vi "LINX - Photocell_to water level.vi"(8 "AI Channel":u8, 11 "Serial Port":refnum<visa-resource-name>) -> (0 "Photocell Value":u8(slide) scale=0.0..15.0)   [LabVIEW 2020]
doc: "Measure light intensity using a photocell."
uses:
  <vilib>/MakerHub/LINX/Public/Utilities/Open Serial.vi
  <vilib>/MakerHub/LINX/LMH-LINX.lvlib
panel:
  out "Loop Rate (Hz)":u32
  in  "Stop Button":bool
  # "Circuit Schematic"
  # "LINX Device Settings"
  # "Photocell Value"
  # "Photocell Example (Serial Interface)\n\nThis example demonstrates how to measure light intensity using a photocell.\n\nInstructions\n1. Select the COM Port associated with the LINX Device.\n2. Select the Analog Channel connected to the photocell.\n3. Click the Run Arrow."
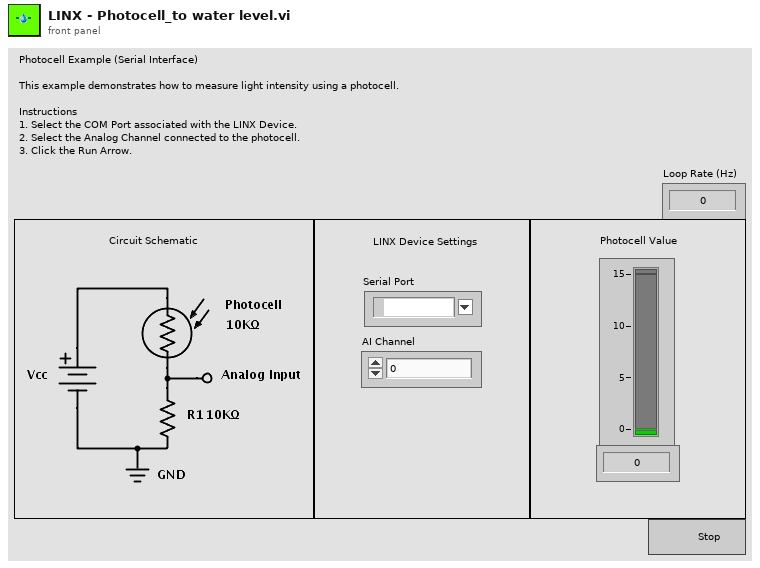
[diagram p1: front panel]
types:
  T1 = typedef "LMH-LINX.lvlib/LINX Ref.ctl" = cluster{"IO":T2, "Interface":T3, "LINX Device Config":T4}
  T2 = typedef "LMH-LINX.lvlib/Platform.ctl" = enum16{"Remote", "Local"}
  T3 = typedef "LMH-LINX.lvlib/Interface.ctl" = enum16{"Serial", "TCP"}
  T4 = typedef "LMH-LINX.lvlib/Device.lvlib/LINX Device Config.ctl" = cluster{"Interface":T3, "COM Port":refnum<visa-resource-name>, "TCP Configuration":T5, "Device Family":u8, "Device ID":u8, "Device Name":string, "TCP Ref":refnum<k5>, "Channels":T6}
  T5 = typedef "LMH-LINX.lvlib/Device.lvlib/TCP Config.ctl" = cluster{"IP Address":string, "Port":u16}
  T6 = typedef "LMH-LINX.lvlib/Channels.ctl" = cluster{"DI":u8[], "DO":u8[], "AI":u8[], "AO":u8[], "PWM":u8[], "QE":u8[], "UART":u8[], "I2C 2":u8[], "SPI":u8[], "CAN":u8[], "Servo":u8[], "AI Ref (V)":dbl, "AI Resolution (Bits)":u8, "AO Ref (V)":dbl, "AO Resolution (Bits)":u8}
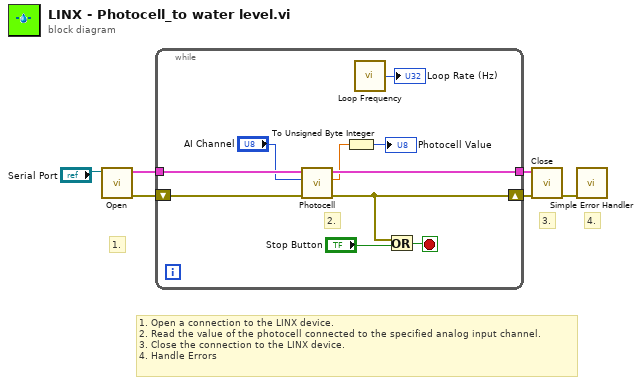
[diagram p0: block diagram]
diagram:
  # "1. Open a connection to the LINX device.\n2. Read the value of the photocell connected to the specified analog input channel.\n3. Close the connection to the LINX device.\n4. Handle Errors"
  # "4."
  # "3."
  # "1."
  n1 = call-poly <vilib>:"Open.vi"("Serial Port"="Serial Port") -> ("Error Out"=w5:errorcluster, "LINX Resource"=w6:T1)  [unwired: 8 in, 1 out]
  n2 = while {
    tunnel: w6 -> [w13]
    tunnel: [w12] -> w4
    shift-right: [w11] -> w3
    shift-left: w5 -> [w10]
    stop <- w16 stop-if-true
    # "2."
    n3 = call <vilib>:"Photocell.vi"("Error In"=w10, "AI Channel"="AI Channel", "LINX Resource"=w13) -> ("Error Out"=w11:errorcluster, "Value (0-100)"=w7:dbl, "LINX Resource"=w12:T1)  [unwired: 6 in]
    n4 = To Unsigned Byte Integer(number=w7) -> (unsigned 8bit integer=→"Photocell Value":u8)
    n5 = call <vilib>:"Loop Frequency.vi"() -> ("Loop Rate (Hz)"=→"Loop Rate (Hz)":u32)
    n6 = Or(x=w11, y="Stop Button") -> (x .or. y?=w16:bool)
  }
  n7 = call <vilib>:"Close.vi"("Error In"=w3, "LINX Resource"=w4) -> ("Error Out"=w1:errorcluster)  [unwired: 9 in]
  n8 = call <vilib>:"Simple Error Handler.vi"("error in (no error)"=w1) -> ()  [unwired: 4 in, 5 out]
